vi "Read Instrument Ini file.vi"(8 "error in (no error)":errorcluster) -> (0 "error out":errorcluster, 1 "Environmental List":string[][](array[string]), 2 "Instrument List":string[][](array[string]), 3 "User List":string[][](array[string]), 4 "# of Instruments":i32, 5 "# of User":i32, 6 "# of Environ":i32)   [LabVIEW 2020, in "Test Framework.lvclass"]
doc: "Reads the instrument ini file and outputs the instrument and reference choices"
uses:
  Test Framework.lvclass
  <vilib>/Utility/config.llb/Read Key (String).vi
  <vilib>/Utility/config.llb/NI_LVConfig.lvlib
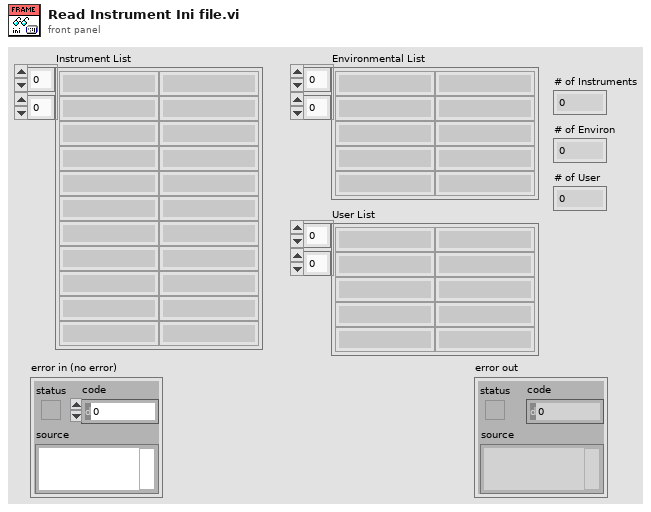
[diagram p1: front panel]
types:
  T1 = typedef "NI_LVConfig.lvlib/Config Data RefNum.ctl" = refnum<k1>
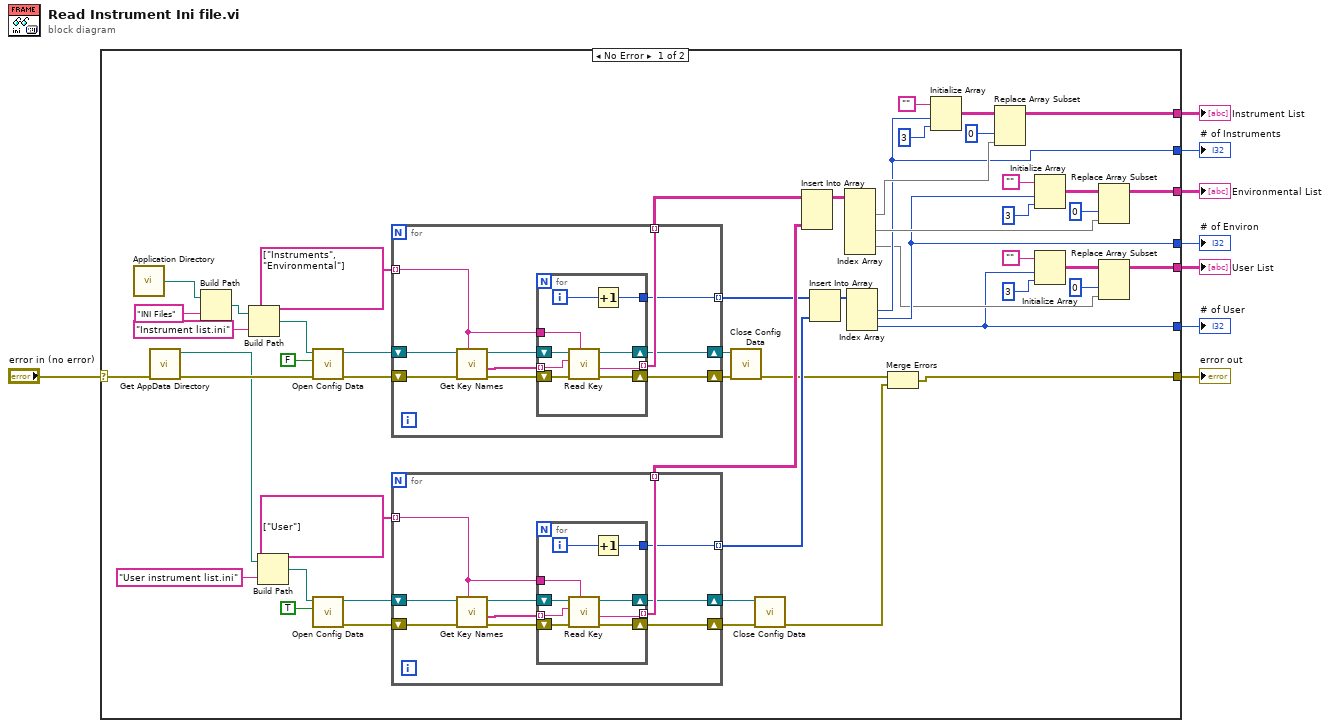
[diagram p0: block diagram]
diagram:
  n1 = case shown="No Error" "error in (no error)" {
    selector: "error in (no error)" -> [w22 w99]
    tunnel: [w9 w99] -> w7
    tunnel: [w41 _] -> w6
    tunnel: [w40 _] -> w5
    tunnel: [w39 _] -> w4
    tunnel: [w38 _] -> w3
    tunnel: [w37 _] -> w1
    tunnel: [w31 _] -> w2
    frame No Error {
      n2 = call <vilib>:"Application Directory.vi"() -> ("Application Directory"=w60:path)
      n3 = call "Get AppData Directory.vi"("Error In"=w22) -> ("Error Out"=w21:errorcluster, "Folder path"=w18:path)  [unwired: 8 in, 1 out]
      n4 = Build Path(base path=w60, name or relative path="INI Files") -> (appended path=w58:path)
      n5 = Build Path(base path=w58, name or relative path="Instrument list.ini") -> (appended path=w56:path)
      n6 = Build Path(base path=w18, name or relative path="User instrument list.ini") -> (appended path=w19:path)
      n7 = call <vilib>:"Open Config Data.vi"("error in (no error)"=w21, "create file if necessary (T)"=FALSE, "configuration file path"=w56) -> ("error out"=w54:errorcluster, "refnum"=w53:T1)  [unwired: 6 in, 1 out]
      n8 = call <vilib>:"Open Config Data.vi"("create file if necessary (T)"=TRUE, "configuration file path"=w19) -> ("error out"=w24:errorcluster, "refnum"=w25:T1)  [unwired: 7 in, 1 out]
      n9 = for {
        tunnel: string[] ["Instruments", "Environmental"] -> [w84] mode=indexing
        tunnel: [w83] -> w17 mode=indexing
        shift-right: [w82] -> w30
        shift-left: w54 -> [w89]
        tunnel: [w81] -> w15 mode=indexing
        shift-right: [w80] -> w29
        shift-left: w53 -> [w88]
        n10 = call <vilib>:"Get Key Names.vi"("section"=w84, "error in (no error)"=w89, "refnum"=w88) -> ("error out"=w87:errorcluster, "key names"=w86:string[], "refnum out"=w85:T1)  [unwired: 5 in, 1 out]
        n11 = for {
          shift-right: [w97] -> w82
          shift-left: w87 -> [w98]
          tunnel: w86 -> [w92] mode=indexing
          tunnel: w84 -> [w95]
          tunnel: [w94] -> w83 mode=indexing
          tunnel: [w90] -> w81
          shift-right: [w93] -> w80
          shift-left: w85 -> [w96]
          i -> [w91]
          n12 = call-poly <vilib>:"Read Key.vi"("section"=w95, "error in (no error)"=w98, "key"=w92, "refnum"=w96) -> ("error out"=w97:errorcluster, "value"=w94:string, "refnum out"=w93:T1)  [unwired: 4 in, 1 out]
          n13 = Increment(x=w91) -> (x+1=w90:i32)
        }
      }
      n14 = for {
        tunnel: string[] ["User"] -> [w65] mode=indexing
        tunnel: [w64] -> w16 mode=indexing
        shift-right: [w63] -> w27
        shift-left: w24 -> [w70]
        tunnel: [w62] -> w14 mode=indexing
        shift-right: [w61] -> w28
        shift-left: w25 -> [w69]
        n15 = call <vilib>:"Get Key Names.vi"("section"=w65, "error in (no error)"=w70, "refnum"=w69) -> ("error out"=w68:errorcluster, "key names"=w67:string[], "refnum out"=w66:T1)  [unwired: 5 in, 1 out]
        n16 = for {
          shift-right: [w78] -> w63
          shift-left: w68 -> [w79]
          tunnel: w67 -> [w73] mode=indexing
          tunnel: w65 -> [w76]
          tunnel: [w75] -> w64 mode=indexing
          tunnel: [w71] -> w62
          shift-right: [w74] -> w61
          shift-left: w66 -> [w77]
          i -> [w72]
          n17 = call-poly <vilib>:"Read Key.vi"("section"=w76, "error in (no error)"=w79, "key"=w73, "refnum"=w77) -> ("error out"=w78:errorcluster, "value"=w75:string, "refnum out"=w74:T1)  [unwired: 4 in, 1 out]
          n18 = Increment(x=w72) -> (x+1=w71:i32)
        }
      }
      n19 = call <vilib>:"Close Config Data.vi"("error in (no error)"=w30, "refnum"=w29) -> ("error out"=w10:errorcluster)  [unwired: 8 in, 1 out]
      n20 = call <vilib>:"Close Config Data.vi"("error in (no error)"=w27, "refnum"=w28) -> ("error out"=w11:errorcluster)  [unwired: 8 in, 1 out]
      n21 = Insert Into Array(array=w17, new element=w16) -> (w12:string[][])  [unwired: 2 in]
      n22 = Insert Into Array(array=w15, new element=w14) -> (w13:i32[])  [unwired: 1 in]
      n23 = Index Array(array=w12) -> (element #1=w43:string[], element #2=w42:string[], element #3=w32:string[])  [unwired: 6 in]
      n24 = Index Array(array=w13) -> (element #1=w39:i32, element #2=w38:i32, element #3=w31:i32)  [unwired: 3 in]
      n25 = Merge Errors(w10, w11) -> (w9:errorcluster)
      n26 = Initialize Array("", w39, 3 ("dimension size")) -> (w50:string[][])
      n27 = Replace Array Subset(array=w50, new element=w43, index (col)=0 ("disabled index (col)")) -> (w41:string[][])  [unwired: 1 in]
      n28 = Initialize Array("", w38, 3 ("dimension size")) -> (w47:string[][])
      n29 = Initialize Array("", w31, 3 ("dimension size")) -> (w34:string[][])
      n30 = Replace Array Subset(array=w47, new element=w42, index (col)=0 ("disabled index (col)")) -> (w40:string[][])  [unwired: 1 in]
      n31 = Replace Array Subset(array=w34, new element=w32, index (col)=0 ("disabled index (col)")) -> (w37:string[][])  [unwired: 1 in]
    }
    frame Error {
    }
  }
  "error out" <- w7
  "Instrument List" <- w6
  "Environmental List" <- w5
  "# of Instruments" <- w4
  "# of Environ" <- w3
  "User List" <- w1
  "# of User" <- w2
